vi "DIAdem Un-Escape Apostrophe.vi"(1 "Escaped String":string) -> (0 "String":string)   [LabVIEW 2011]
doc: "Encodes characters in URL format, replacing all characters except for alphanumeric and underscore with %xx, where xx is the hexadecimal value of the character."
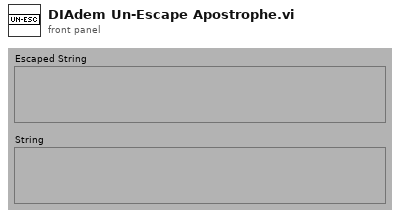
[diagram p1: front panel]
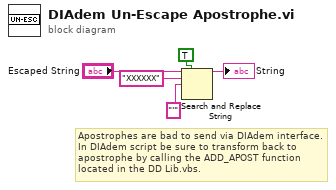
[diagram p0: block diagram]
diagram:
  # "Apostrophes are bad to send via DIAdem interface.\nIn DIAdem script be sure to transform back to\napostrophe by calling the ADD_APOST function\nlocated in the DD Lib.vbs."
  n1 = Search and Replace String(replace all?=TRUE ("replace all? (F)"), input string="Escaped String", search string="XXXXXX", replace string="'" ("replace string (\"\")")) -> (result string=→"String":string)  [unwired: 1 in, 6 out]
